vi "Reject invalid speed data.vi"(9 "Funct data structure":bool, 11 "Spreadsheet data":string[][](array[string])) -> (1 "Valid speed data":dbl[](array[numeric]), 2 "Original number of points":i32, 3 "Valid speed data table":string[][](array[string]))   [LabVIEW 2013]
uses:
  Typedefs/Test header stats cluster.ctl
  Program Files (x86)/National Instruments/LabVIEW 2013/user.lib/_OpenG.lib/array/array.llb/Conditional Auto-Indexing Tunnel (DBL)__ogtk.vi
panel:
  out "Difference (points)":i32
  out "Timestamps length (ms)":dbl
  out "Loaded timestamps (ms)":dbl[](array[numeric]) format="%#_6f"
  out "Acquisition time unknown":bool
  out "Experiment Header's values":T1
  out "Valid timestamps (ms)":dbl[](array[numeric])
  out "Output number of points":i32
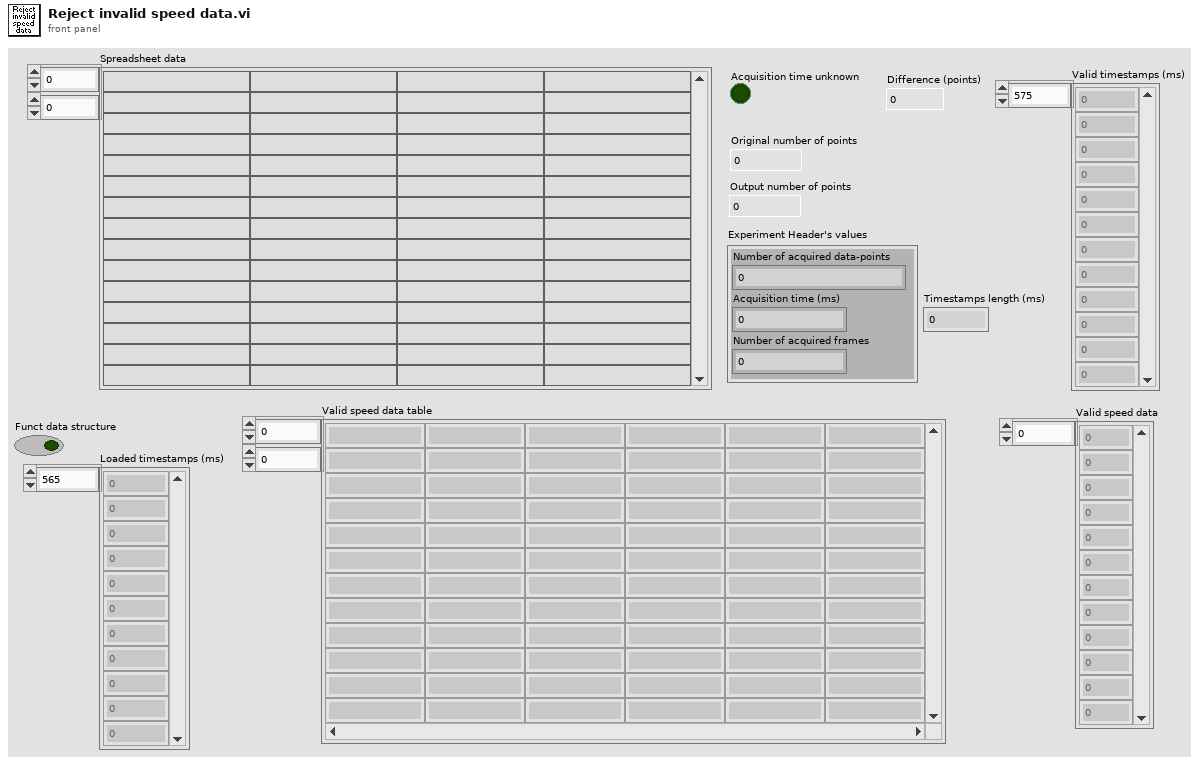
[diagram p1: front panel]
types:
  T1 = typedef "Test header stats cluster.ctl" = cluster{"Number of acquired data-points":dbl, "Acquisition time (ms)":dbl, "Number of acquired frames":dbl}
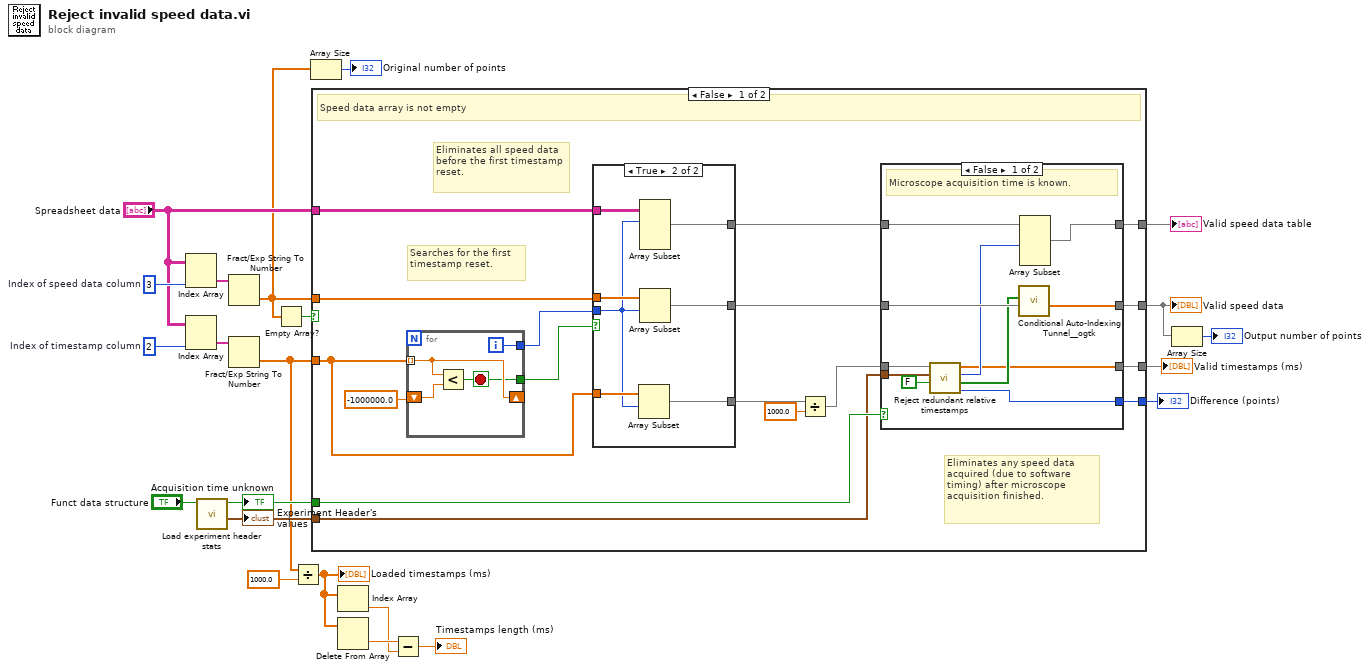
[diagram p0: block diagram]
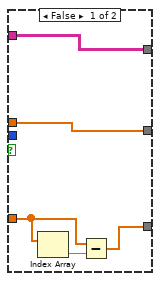
[diagram p3: hidden frame]
diagram:
  w18 = 2  # Index of timestamp column
  w20 = 3  # Index of speed data column
  n1 = Index Array(array="Spreadsheet data", index (col)=w20) -> (element=w21:string[])  [unwired: 1 in]
  n2 = Index Array(array="Spreadsheet data", index (col)=w18) -> (element=w17:string[])  [unwired: 1 in]
  n3 = call "Load experiment header stats.vi"("Funct data structure"="Funct data structure") -> ("Experiment Header's Statistics"=w10:T1, "Acquisition time unknown"=w9:bool)  [unwired: 9 in]
  "Experiment Header's values" <- w10
  "Acquisition time unknown" <- w9
  n4 = Fract/Exp String To Number(string=w21) -> (number=w8:dbl[])  [unwired: 3 in, 1 out]
  n5 = Fract/Exp String To Number(string=w17) -> (number=w6:dbl[])  [unwired: 3 in, 1 out]
  n6 = Empty Array?(array=w8) -> (empty?=w22:bool)
  n7 = Divide(x=w6, y=1000.0) -> (x/y=w5:dbl[])
  "Loaded timestamps (ms)" <- w5
  n8 = Array Size(array=w8) -> (size(s)=→"Original number of points":i32)
  n9 = case shown="False" w22 {
    tunnel: w8 -> [w38 w72]
    tunnel: [w36 w72] -> w12
    tunnel: "Spreadsheet data" -> [w33 w71]
    tunnel: [w31 w71] -> w19
    tunnel: w6 -> [w30 w70]
    tunnel: w10 -> [w25 _]
    tunnel: w9 -> [w27 _]
    tunnel: [w24 w70] -> w11
    tunnel: [w23 _] -> w1
    frame False {
      # "Eliminates any speed data acquired (due to software timing) after microscope acquisition finished."
      # "Eliminates all speed data before the first timestamp reset."
      # "Searches for the first timestamp reset."
      # "Speed data array is not empty"
      n10 = for {
        tunnel: w30 -> [w69] mode=indexing
        shift-right: [w69] -> _
        shift-left: -1000000.0 ("String") -> [w68]
        tunnel: [w67] -> w34
        tunnel: [w66] -> w35
        i -> [w67]
        stop <- w66 stop-if-true
        n11 = Less?(x=w69, y=w68) -> (x < y?=w66:bool)
      }
      n12 = case shown="True" w35 {
        tunnel: w38 -> [w57 w65]
        tunnel: w34 -> [_ w59]
        tunnel: [w57 w64] -> w37
        tunnel: w33 -> [w58 w63]
        tunnel: [w58 w62] -> w32
        tunnel: w30 -> [w55 w61]
        tunnel: [w54 w60] -> w29
        frame False {
          n13 = Index Array(array=w55) -> (element=w56:dbl)  [unwired: 1 in]
          n14 = Subtract(x=w55, y=w56) -> (x-y=w54:dbl[])
        }
        frame True {
          n15 = Array Subset(array=w61, index=w59) -> (w60:dbl[])  [unwired: 1 in]
          n16 = Array Subset "Array Subset"(array=w63, index (row)=w59) -> (w62:string[][])  [unwired: 3 in]
          n17 = Array Subset(array=w65, index=w59) -> (w64:dbl[])  [unwired: 1 in]
        }
      }
      n18 = Divide(x=w29, y=1000.0) -> (x/y=w26:dbl[])
      n19 = case shown="False" w27 {
        tunnel: w37 -> [w50 w53]
        tunnel: [w49 w53] -> w36
        tunnel: [w47 w52] -> w31
        tunnel: w32 -> [w48 w52]
        tunnel: w26 -> [w44 w51]
        tunnel: w25 -> [w43 _]
        tunnel: [w42 w51] -> w24
        tunnel: [w40 _] -> w23
        frame False {
          # "Microscope acquisition time is known."
          n20 = call "Reject redundant relative timestamps.vi"("Acquisition time unknown"=FALSE, "Experiment Header's Statistics"=w43, "Frame relative times array"=w44) -> ("Difference (points)"=w40:i32, "Elements to keep"=w45:bool[], "Number of elements to keep"=w46:i32, "Frame relative times array"=w42:dbl[])  [unwired: 5 in]
          n21 = call-poly "Conditional Auto-Indexing Tunnel__ogtk.vi"("Array in"=w50, "Elements to keep"=w45) -> ("Filtered Array out"=w49:dbl[])  [unwired: 5 in]
          n22 = Array Subset(array=w48, length (row)=w46) -> (w47:string[][])  [unwired: 3 in]
        }
        frame True {
          # "Microscope acquisition time unknown."
        }
      }
    }
    frame True {
      # "Empty speed data array"
    }
  }
  "Valid speed data" <- w12
  "Valid speed data table" <- w19
  "Valid timestamps (ms)" <- w11
  "Difference (points)" <- w1
  n23 = Index Array(array=w5) -> (element=w3:dbl)  [unwired: 1 in]
  n24 = Delete From Array(array=w5) -> (deleted portion=w4:dbl)  [unwired: 2 in, 1 out]
  n25 = Subtract(x=w4, y=w3) -> (x-y=→"Timestamps length (ms)":dbl)
  n26 = Array Size(array=w12) -> (size(s)=→"Output number of points":i32)
